vi "depth rate 2016.vi"(1 "Depth Last":dbl format="%.2f", 2 "Depth Current":dbl format="%.2f", 3 "Time Last":dbl, 4 "Time Current":dbl) -> (0 "Depth Rate":dbl format="%.2f")   [LabVIEW 2016]
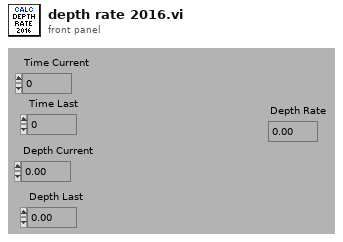
[diagram p1: front panel]
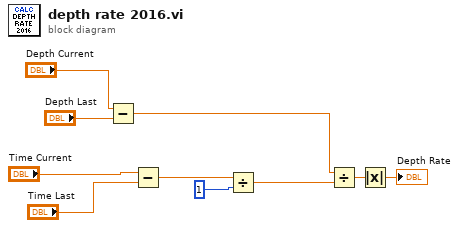
[diagram p0: block diagram]
diagram:
  n1 = Subtract(x="Depth Current", y="Depth Last") -> (x-y=w8:dbl)
  n2 = Subtract(x="Time Current", y="Time Last") -> (x-y=w2:dbl)
  n3 = Divide(x=w2, y=1) -> (x/y=w3:dbl)
  n4 = Divide(x=w8, y=w3) -> (x/y=w5:dbl)
  n5 = Absolute Value(x=w5) -> (abs(x)=→"Depth Rate":dbl)
